vi "Create_Trajectory_Get_Field_Info.vi"(11 "Field Selector":string) -> (2 "File":string, 3 "input cluster":T1)   [LabVIEW 2019]
uses:
  TrajectoryUtils_Field_Info.ctl
  <vilib>/Utility/config.llb/Read Key (String).vi
  <vilib>/Utility/config.llb/Read Key (I32).vi
  <vilib>/Utility/config.llb/Read Key (Double).vi
  <vilib>/Utility/config.llb/NI_LVConfig.lvlib
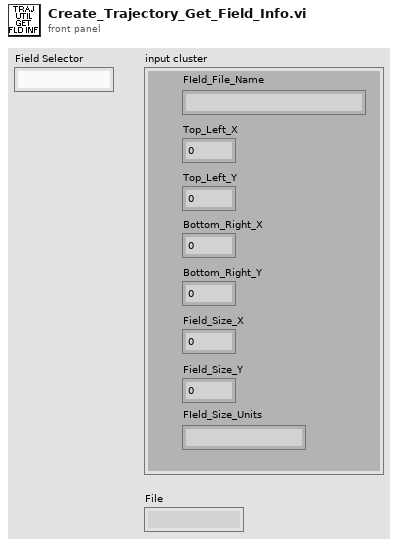
[diagram p1: front panel]
types:
  T1 = typedef "TrajectoryUtils_Field_Info.ctl" = cluster{"FIeld_File_Name":string, "Top_Left_X":i32, "Top_Left_Y":i32, "Bottom_Right_X":i32, "Bottom_Right_Y":i32, "Field_Size_X":dbl, "Field_Size_Y":dbl, "FIeld_Size_Units":string}
  T2 = typedef "NI_LVConfig.lvlib/Config Data RefNum.ctl" = refnum<k1>
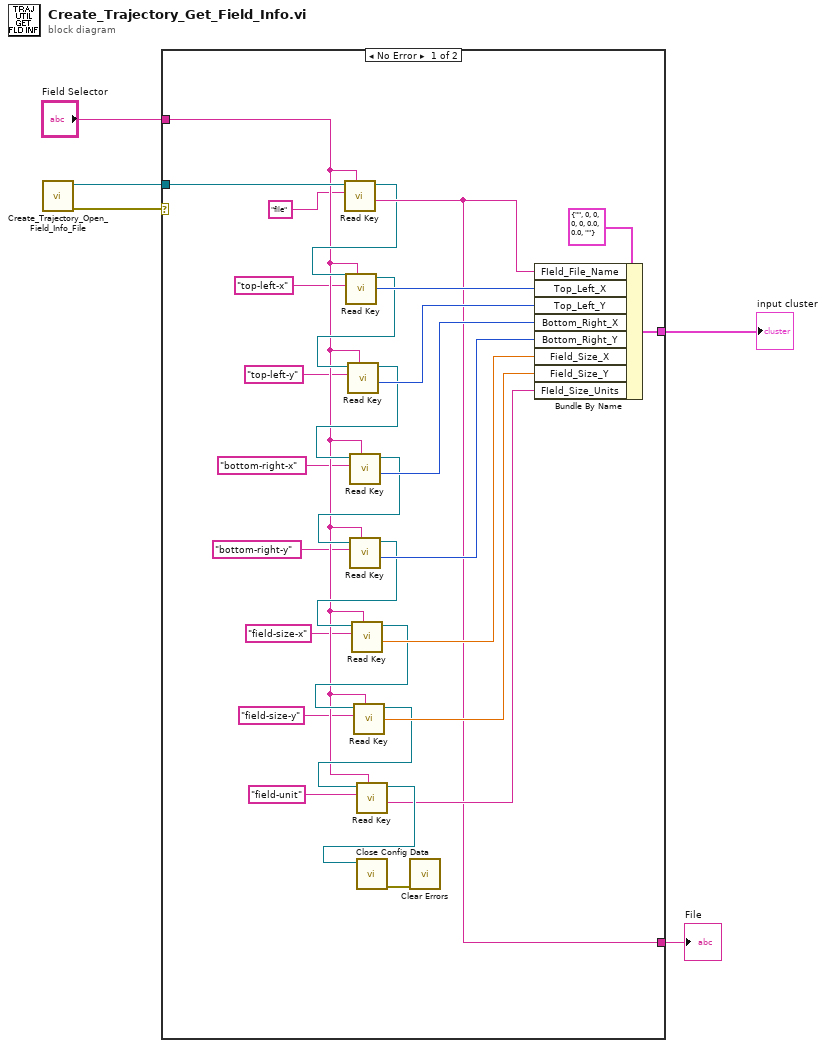
[diagram p0: block diagram]
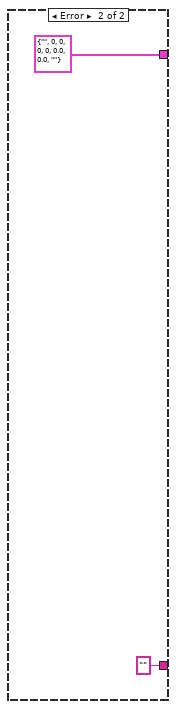
[diagram p2: hidden frame]
diagram:
  n1 = call "Create_Trajectory_Open_Field_Info_File.vi"() -> ("error out"=w1:errorcluster, "Refnum out"=w3:T2)  [unwired: 10 in]
  n2 = case shown="No Error" w1 {
    tunnel: [w26 T1 {"FIeld_File_Name"="", "Top_Left_X"=0, "Top_Left_Y"=0, "Bottom_Right_X"=0, "Bottom_Right_Y"=0, "Field_Size_X"=0.0, "Field_Size_Y"=0.0, "FIeld_Size_Units"=""} ("input cluster")] -> w5
    tunnel: [w25 "" ("value")] -> w4
    tunnel: w3 -> [w16 _]
    tunnel: "Field Selector" -> [w15 _]
    frame No Error {
      n3 = call-poly <vilib>:"Read Key.vi"("section"=w15, "key"="file", "refnum"=w16) -> ("value"=w25:string, "refnum out"=w17:T2)  [unwired: 5 in, 2 out]
      n4 = call-poly <vilib>:"Read Key.vi"("section"=w15, "key"="top-left-x", "refnum"=w17) -> ("value"=w30:i32, "refnum out"=w18:T2)  [unwired: 5 in, 2 out]
      n5 = call-poly <vilib>:"Read Key.vi"("section"=w15, "key"="top-left-y", "refnum"=w18) -> ("value"=w27:i32, "refnum out"=w19:T2)  [unwired: 5 in, 2 out]
      n6 = call-poly <vilib>:"Read Key.vi"("section"=w15, "key"="bottom-right-x", "refnum"=w19) -> ("value"=w31:i32, "refnum out"=w20:T2)  [unwired: 5 in, 2 out]
      n7 = call-poly <vilib>:"Read Key.vi"("section"=w15, "key"="bottom-right-y", "refnum"=w20) -> ("value"=w28:i32, "refnum out"=w21:T2)  [unwired: 5 in, 2 out]
      n8 = call-poly <vilib>:"Read Key.vi"("section"=w15, "key"="field-size-x", "refnum"=w21) -> ("value"=w29:dbl, "refnum out"=w22:T2)  [unwired: 5 in, 2 out]
      n9 = call-poly <vilib>:"Read Key.vi"("section"=w15, "key"="field-size-y", "refnum"=w22) -> ("value"=w32:dbl, "refnum out"=w23:T2)  [unwired: 5 in, 2 out]
      n10 = call-poly <vilib>:"Read Key.vi"("section"=w15, "key"="field-unit", "refnum"=w23) -> ("value"=w33:string, "refnum out"=w34:T2)  [unwired: 5 in, 2 out]
      n11 = call <vilib>:"Close Config Data.vi"("refnum"=w34) -> ("error out"=w6:errorcluster)  [unwired: 9 in, 1 out]
      n12 = call <vilib>:"Clear Errors.vi"("error in (no error)"=w6) -> ()  [unwired: 5 in, 2 out]
      n13 = Bundle By Name(cluster=T1 {"FIeld_File_Name"="", "Top_Left_X"=0, "Top_Left_Y"=0, "Bottom_Right_X"=0, "Bottom_Right_Y"=0, "Field_Size_X"=0.0, "Field_Size_Y"=0.0, "FIeld_Size_Units"=""} ("input cluster"), "FIeld_File_Name"=w25, "Top_Left_X"=w30, "Top_Left_Y"=w27, "Bottom_Right_X"=w31, "Bottom_Right_Y"=w28, "Field_Size_X"=w29, "Field_Size_Y"=w32, "FIeld_Size_Units"=w33) -> (w26:T1)
    }
    frame Error {
    }
  }
  "input cluster" <- w5
  "File" <- w4
